vi "IDS_rt_getAafAttenuation.vi"(0 "deviceHandle":i32, 1 "error in (no error)":errorcluster) -> (2 "deviceHandle out":i32, 3 "Attenuation":i32, 4 "error out":errorcluster)   [LabVIEW 2016]
doc: "int IDS_DLL IDS_rt_getResolutionSinCos(int32_t * resolution);"
uses:
  G:/SCMOperations/Share/SEN/Produkt Information/04 IDS/Software/00_IDS Firmware Releases/IDS_Firmware_V1.9.1/06_LabVIEW/IDS Legacy VIs (DLL-based)/dlls/ids-library.dll
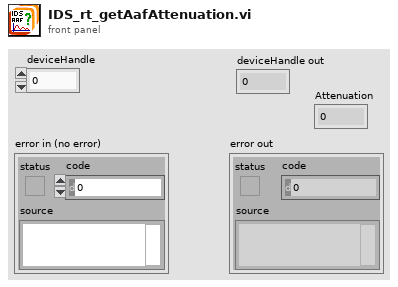
[diagram p1: front panel]
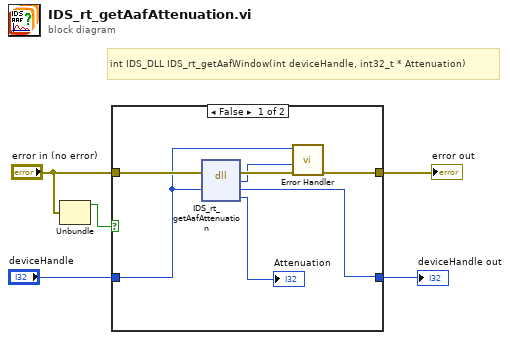
[diagram p0: block diagram]
diagram:
  # "int IDS_DLL IDS_rt_getAafWindow(int deviceHandle, int32_t * Attenuation)"
  n1 = Unbundle("error in (no error)") -> ("status"=w1:bool)  [unwired: 2 out]
  n2 = case shown="False" w1 {
    tunnel: "error in (no error)" -> [w11 w14]
    tunnel: [w12 w14] -> w5
    tunnel: "deviceHandle" -> [w7 w13]
    tunnel: [w9 w13] -> w3
    frame False {
      n3 = dll-call lib="G:/SCMOperations/Share/SEN/Produkt Information/04 IDS/Software/00_IDS Firmware Releases/IDS_Firmware_V1.9.1/06_LabVIEW/IDS Legacy VIs (DLL-based)/dlls/ids-library.dll" fn="IDS_rt_getAafAttenuation"(error in=w11, "deviceHandle"=w7) -> (error out=w10:errorcluster, "return type"=w8:i32, "deviceHandle"=w9:i32, "Attenuation"=→"Attenuation":i32)  [unwired: 3 in, 1 out]
      n4 = call "Error Handler.vi"("error in (no error)"=w10, "error code"=w8, "deviceHandle"=w7) -> ("error out"=w12:errorcluster)  [unwired: 7 in, 1 out]
    }
    frame True {
    }
  }
  "error out" <- w5
  "deviceHandle out" <- w3
